vi "Misc. 1.vi"() -> ()   [LabVIEW 2017]
uses:
  <vilib>/Math Plots/3D Math Plots/3D Bar/3D Bar XCtrl/3D Bar.xctl
  <vilib>/Math Plots/3D Math Plots/3D Bar/3D Bar Datatype/Public/Plot Helper (Matrix).vi
  <vilib>/Math Plots/3D Math Plots/3D Bar/3D Bar Datatype/3D Bar Datatype.lvclass
panel:
  in  "dimension size":i32=3
  in  "Boolean":bool
  out "output array":dbl[][](array[numeric])
  out "appended array 2":dbl[](array[numeric])
  out "3D Bar":refnum<class "3D Plot Datatype.lvclass">[](xcontrol)
  out "appended array":dbl[](array[numeric])
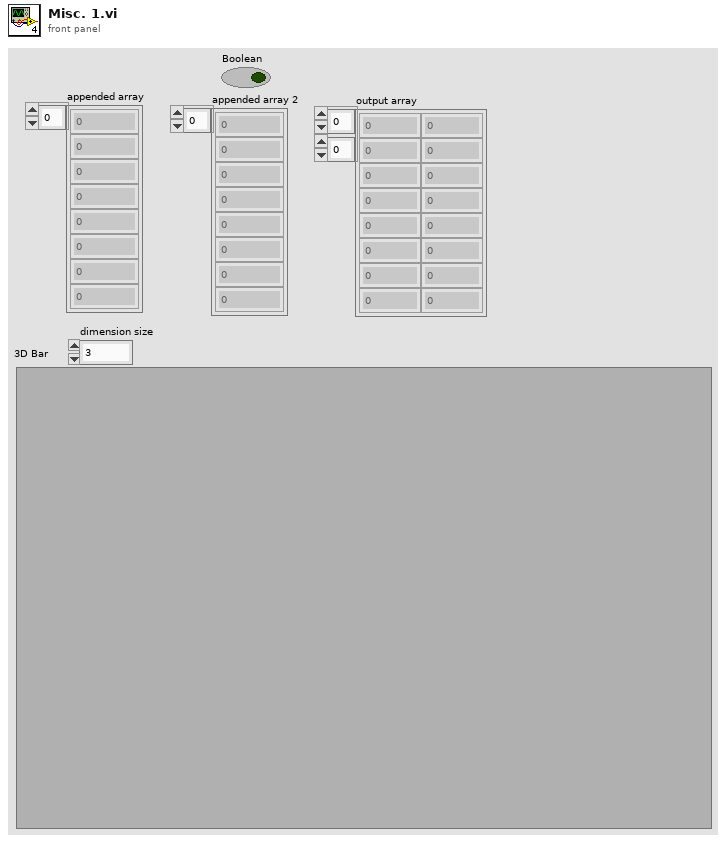
[diagram p1: front panel]
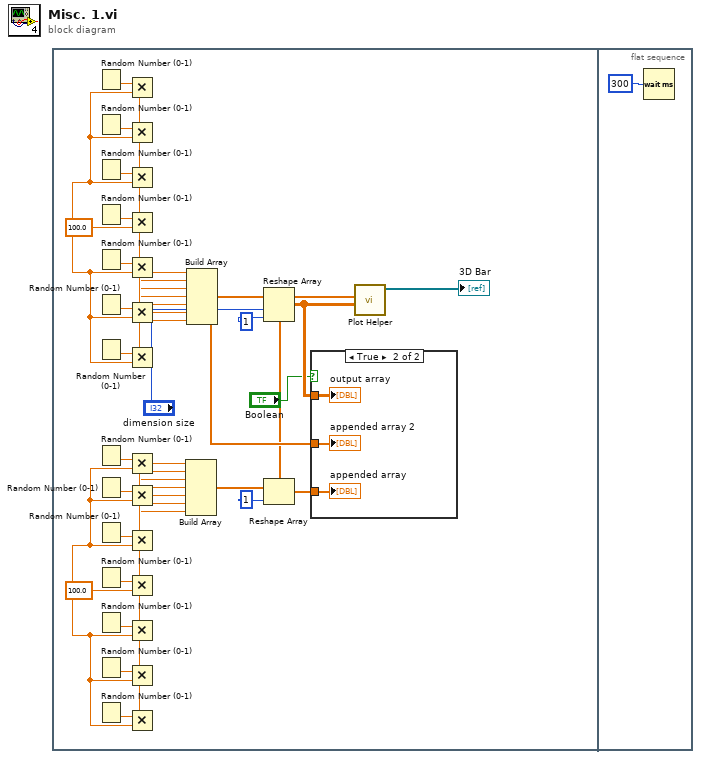
[diagram p0: block diagram]
diagram:
  n1 = flat-sequence {
    frame #0 {
      w23 = 100.0 ("y")
      w25 = 100.0 ("y")
      n2 = Random Number (0-1)() -> (number: 0 to 1=w9:dbl)
      n3 = Random Number (0-1)() -> (number: 0 to 1=w11:dbl)
      n4 = Random Number (0-1)() -> (number: 0 to 1=w13:dbl)
      n5 = Random Number (0-1)() -> (number: 0 to 1=w14:dbl)
      n6 = Random Number (0-1)() -> (number: 0 to 1=w17:dbl)
      n7 = Random Number (0-1)() -> (number: 0 to 1=w19:dbl)
      n8 = Random Number (0-1)() -> (number: 0 to 1=w21:dbl)
      n9 = Random Number (0-1)() -> (number: 0 to 1=w39:dbl)
      n10 = Random Number (0-1)() -> (number: 0 to 1=w37:dbl)
      n11 = Random Number (0-1)() -> (number: 0 to 1=w35:dbl)
      n12 = Random Number (0-1)() -> (number: 0 to 1=w34:dbl)
      n13 = Random Number (0-1)() -> (number: 0 to 1=w31:dbl)
      n14 = Random Number (0-1)() -> (number: 0 to 1=w29:dbl)
      n15 = Random Number (0-1)() -> (number: 0 to 1=w27:dbl)
      n16 = Multiply(x=w9, y=w23) -> (x*y=w10:dbl)
      n17 = Multiply(x=w11, y=w23) -> (x*y=w12:dbl)
      n18 = Multiply(x=w13, y=w23) -> (x*y=w15:dbl)
      n19 = Multiply(x=w14, y=w23) -> (x*y=w16:dbl)
      n20 = Multiply(x=w17, y=w23) -> (x*y=w18:dbl)
      n21 = Multiply(x=w19, y=w23) -> (x*y=w20:dbl)
      n22 = Multiply(x=w21, y=w23) -> (x*y=w22:dbl)
      n23 = Multiply(x=w39, y=w25) -> (x*y=w38:dbl)
      n24 = Multiply(x=w37, y=w25) -> (x*y=w36:dbl)
      n25 = Multiply(x=w35, y=w25) -> (x*y=w33:dbl)
      n26 = Multiply(x=w34, y=w25) -> (x*y=w32:dbl)
      n27 = Multiply(x=w31, y=w25) -> (x*y=w30:dbl)
      n28 = Multiply(x=w29, y=w25) -> (x*y=w28:dbl)
      n29 = Multiply(x=w27, y=w25) -> (x*y=w26:dbl)
      n30 = Build Array(w38, w36, w33, w32, w30, w28, w26) -> (w3:dbl[])
      n31 = Build Array(w10, w12, w15, w16, w18, w20, w22) -> (w8:dbl[])
      n32 = Reshape Array(w8, "dimension size", 1 ("dimension size")) -> (w5:dbl[][])
      n33 = Reshape Array(w3, 1 ("dimension size")) -> (w1:dbl[])
      n34 = case shown="True" "Boolean" {
        tunnel: w8 -> [_ w42]
        tunnel: w5 -> [_ w41]
        tunnel: w1 -> [_ w40]
        frame False {
        }
        frame True {
          "appended array" <- w40
          "appended array 2" <- w42
          "output array" <- w41
        }
      }
      n35 = call-poly <vilib>:"Plot Helper.vi"("z matrix"=w5, "y vector"=w1) -> ("3D Plot lvclass Array out"=→"3D Bar":refnum<class "3D Plot Datatype.lvclass">[])  [unwired: 1 in, 8 out]
    }
    frame #1 {
      n36 = Wait (ms)(milliseconds to wait=u32 300) -> ()  [unwired: 1 out]
    }
  }
